vi "Get Server Stop UE.vi"(11 "OOP Server in":refnum<class "server1.lvclass">) -> (2 "Server Stop UE":refnum<user-event>, 3 "OOP Server out":refnum<class "server1.lvclass">)   [LabVIEW 2020, in "server1.lvlib" / "server1.lvclass"]
uses:
  server1.lvclass
  server1.lvclass/server1.ctl
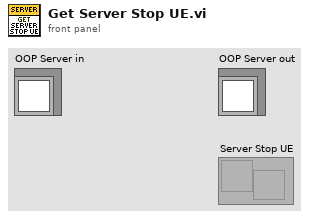
[diagram p1: front panel]
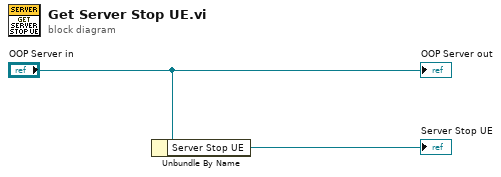
[diagram p0: block diagram]
diagram:
  n1 = Unbundle By Name("OOP Server in") -> ("Server Stop UE"=→"Server Stop UE":refnum<user-event>)
  "OOP Server out" <- "OOP Server in"
